vi "VI_GetChListFromFPElement.vi"(8 "error in (no error)":errorcluster, 11 "ChList_Ref In":refnum<vi>) -> (0 "error out":errorcluster, 1 "Channel IDs":string[](array[string]), 2 "Channel Names":string[](array[string]), 3 "ChList_Ref Out":refnum<vi>)   [LabVIEW 2018]
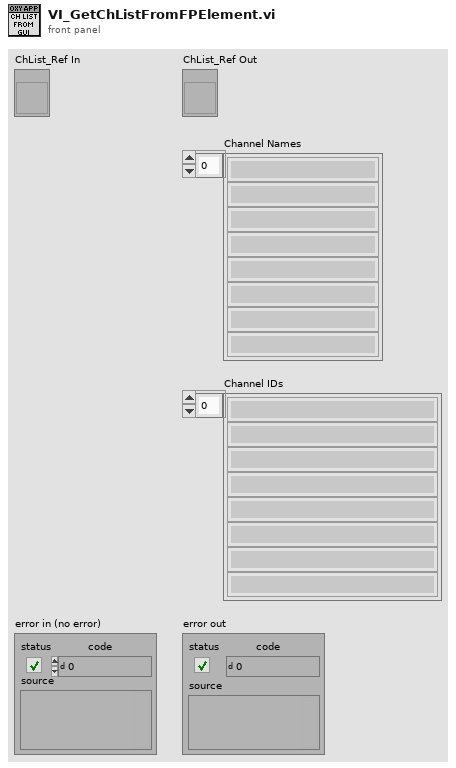
[diagram p1: front panel]
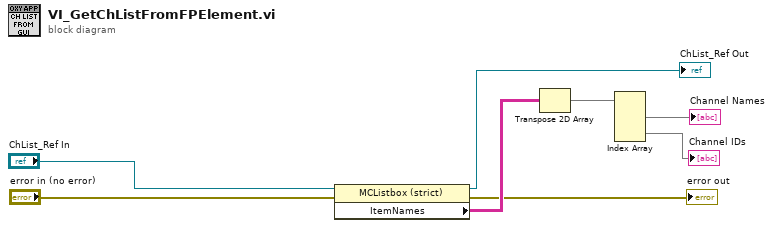
[diagram p0: block diagram]
diagram:
  n1 = property class="MCListbox (strict)"(reference="ChList_Ref In", error in="error in (no error)") -> (reference out=→"ChList_Ref Out":refnum<vi>, error out=→"error out":errorcluster, "ItemNames"=w7:string[][])
  n2 = Transpose 2D Array(2D array=w7) -> (transposed array=w6:string[][])
  n3 = Index Array(array=w6) -> (element #1=→"Channel Names":string[], element #2=→"Channel IDs":string[])  [unwired: 4 in]
